vi "downloadUpdate.vi"(8 "error in (no error)":errorcluster) -> (0 "error out":errorcluster, 3 "appended path":path)   [LabVIEW 2013, in "main.lvlib"]
uses:
  main.lvlib
  <vilib>/httpClient/LabVIEWHTTPClient.lvlib
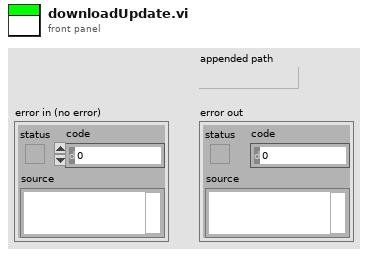
[diagram p1: front panel]
types:
  T1 = typedef "LabVIEWHTTPClient.lvlib/ClientHandle.ctl" = refnum<k1>
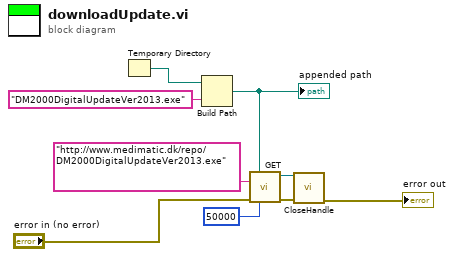
[diagram p0: block diagram]
diagram:
  n1 = Temporary Directory() -> (w2:path)
  n2 = Build Path(base path=w2, name or relative path="DM2000DigitalUpdateVer2013.exe") -> (appended path=w8:path)
  "appended path" <- w8
  n3 = call <vilib>:"GET.vi"("output file"=w8, "url"="http://www.medimatic.dk/repo/DM2000DigitalUpdateVer2013.exe", "error in (no error)"="error in (no error)", "timeout (10000)"=50000) -> ("client handle out"=w5:T1, "error out"=w4:errorcluster)  [unwired: 8 in, 2 out]
  n4 = call <vilib>:"CloseHandle.vi"("client handle"=w5, "error in (no error)"=w4) -> ("error out"=→"error out":errorcluster)  [unwired: 13 in]
